vi "test_Read Analog PWM In.vi"(8 "error in (no error)":errorcluster, 11 "TestCase in":refnum<class "FPGA Addon Speciality IO Tests.lvclass">=refnum) -> (0 "error out":errorcluster, 3 "TestCase out":refnum<class "FPGA Addon Speciality IO Tests.lvclass">)   [LabVIEW 2026, in "FPGA Addon Speciality IO Tests.lvclass"]
uses:
  FPGA Addon Speciality IO Tests.lvclass
  FPGA Addon Test Class/FPGA Addon Test Class.lvclass
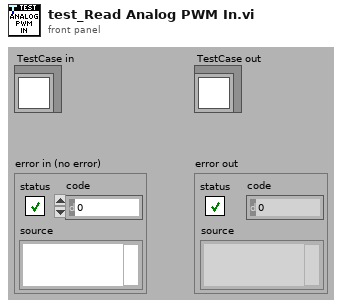
[diagram p1: front panel]
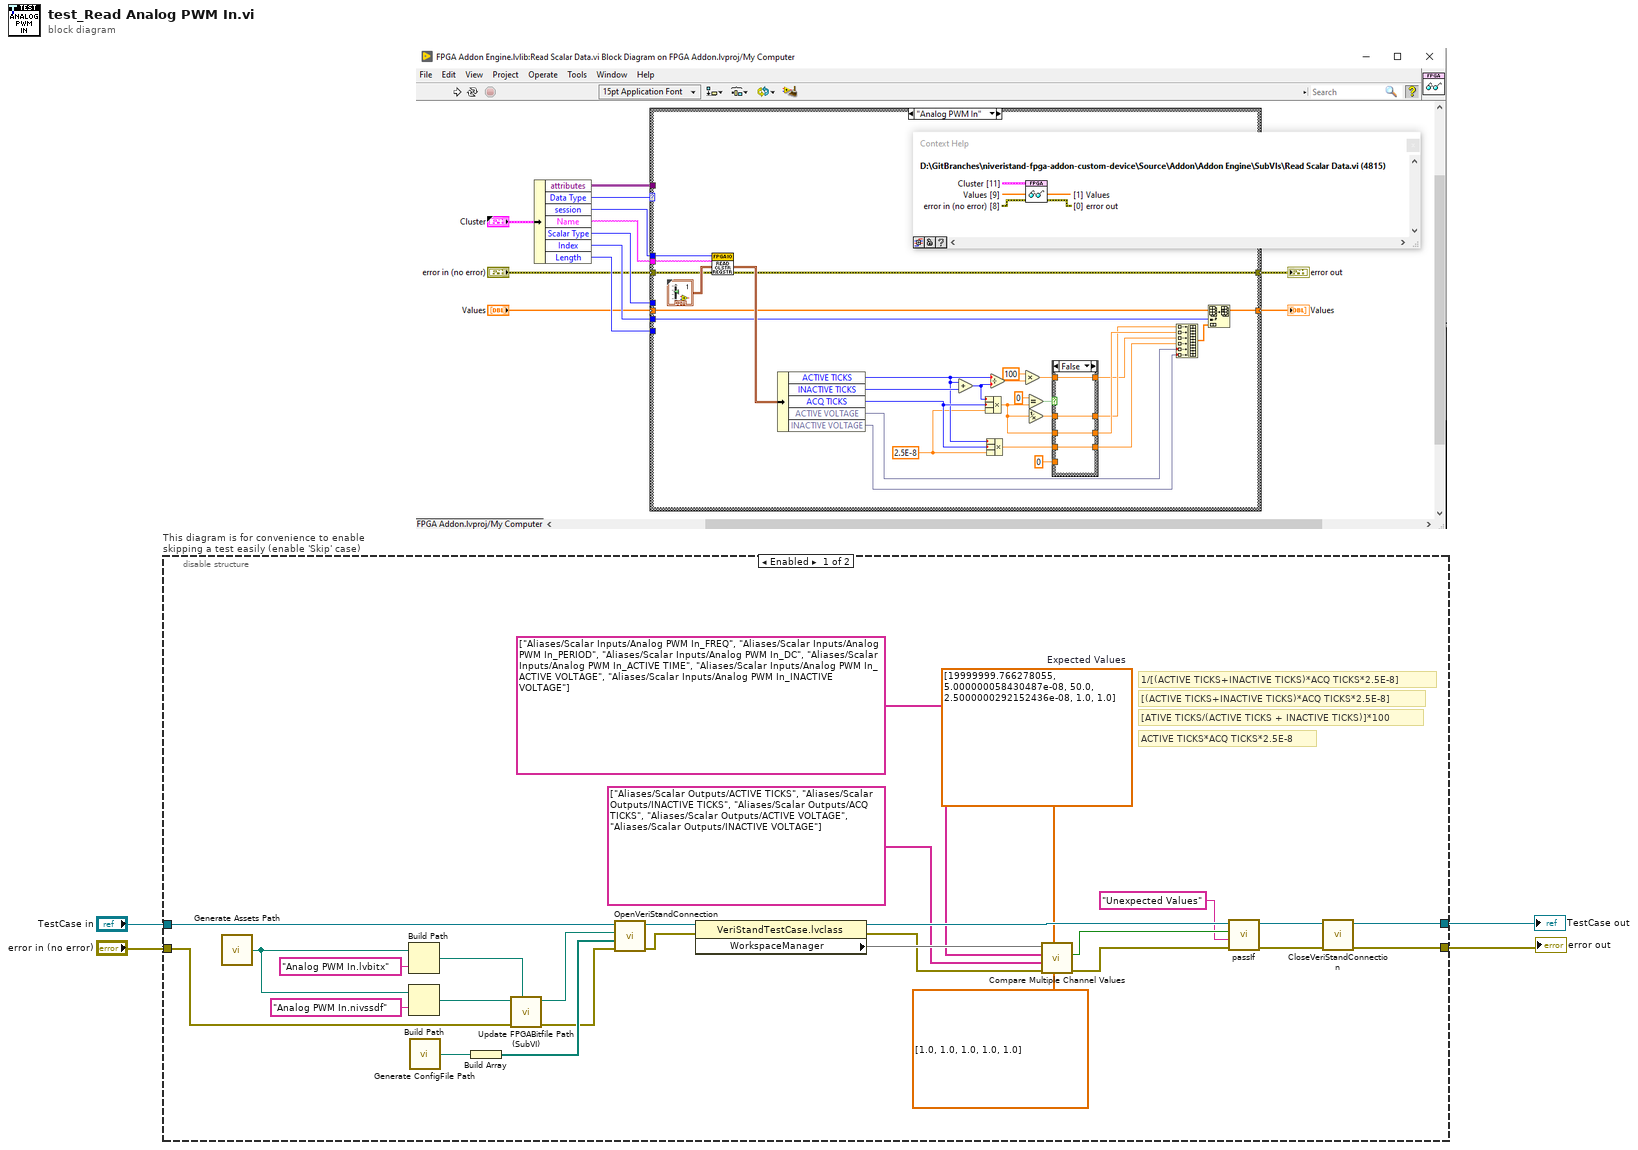
[diagram p0: block diagram]
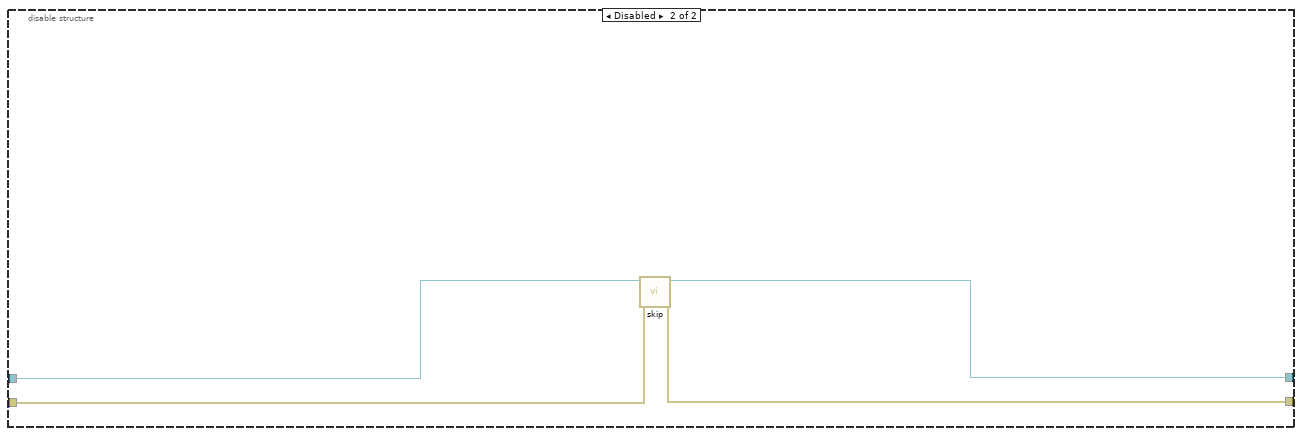
[diagram p2: hidden frame]
diagram:
  n1 = disable-structure "This diagram is for convenience to enable skipping a test easily (enable 'Skip' case)" shown="Enabled" {
    disable-tunnel: "TestCase in" -> [w29 w35]
    disable-tunnel: [w26 w33] -> w1
    disable-tunnel: [w27 w34] -> w3
    disable-tunnel: "error in (no error)" -> [w7 w32]
    frame Enabled {
      w16 = dbl[] [19999999.766278055, 5.000000058430487e-08, 50.0, 2.5000000292152436e-08, 1.0, 1.0]  # Expected Values
      # "ACTIVE TICKS*ACQ TICKS*2.5E-8"
      # "[ATIVE TICKS/(ACTIVE TICKS + INACTIVE TICKS)]*100"
      # "[(ACTIVE TICKS+INACTIVE TICKS)*ACQ TICKS*2.5E-8]"
      # "1/[(ACTIVE TICKS+INACTIVE TICKS)*ACQ TICKS*2.5E-8]"
      n2 = call "Generate Assets Path.vi"() -> ("Assets path"=w12:path)
      n3 = Build Path(base path=w12, name or relative path="Analog PWM In.lvbitx") -> (appended path=w9:path)
      n4 = Build Path(base path=w12, name or relative path="Analog PWM In.nivssdf") -> (appended path=w8:path)
      n5 = call "Generate ConfigFile Path.vi"() -> ("ConfigFile path"=w25:path)
      n6 = Build Array(w25) -> (w28:path[])
      n7 = call "Update FPGABitfile Path (SubVI).vi"("Bitfile Path"=w9, "error in (no error)"=w7, "System Definition path in"=w8) -> ("error out"=w6:errorcluster, "System Definition path out"=w5:path)  [unwired: 7 in]
      n8 = call-dynamic "OpenVeriStandConnection.vi"("error in (no error)"=w6, "overrides files"=w28, "System Definition File"=w5, "VeriStand Test Case in"=w29) -> ("error out"=w31:errorcluster, "VeriStand Test Case out"=w30:refnum<class "VeriStandTestCase.lvclass">)  [unwired: 5 in, 1 out]
      n9 = property class="VeriStandTestCase.lvclass"(reference=w30, error in=w31) -> (reference out=w24:refnum<class "VeriStandTestCase.lvclass">, error out=w20:errorcluster, "WorkspaceManager"=w21)
      n10 = call "Compare Multiple Channel Values.vi"("Values"=dbl[] [1.0, 1.0, 1.0, 1.0, 1.0], "Expected Values"=w16, "error in (no error)"=w20, "Scalar Outputs"=string[] ["Aliases/Scalar Outputs/ACTIVE TICKS", "Aliases/Scalar Outputs/INACTIVE TICKS", "Aliases/Scalar Outputs/ACQ TICKS", "Aliases/Scalar Outputs/ACTIVE VOLTAGE", "Aliases/Scalar Outputs/INACTIVE VOLTAGE"] ("Channels"), "Scalar Inputs"=string[] ["Aliases/Scalar Inputs/Analog PWM In_FREQ", "Aliases/Scalar Inputs/Analog PWM In_PERIOD", "Aliases/Scalar Inputs/Analog PWM In_DC", "Aliases/Scalar Inputs/Analog PWM In_ACTIVE TIME", "Aliases/Scalar Inputs/Analog PWM In_ACTIVE VOLTAGE", "Aliases/Scalar Inputs/Analog PWM In_INACTIVE VOLTAGE"] ("Channels"), ".NET Refnum in"=w21) -> ("error out"=w15:errorcluster, "Equals?"=w14:bool)  [unwired: 4 in]
      n11 = call-dynamic "passIf.vi"("error in (no error)"=w15, "message (\"\")"="Unexpected Values" ("message (\"\")"), "pass"=w14, "TestCase in"=w24) -> ("error out"=w22:errorcluster, "TestCase out"=w23:refnum<class "FPGA Addon Speciality IO Tests.lvclass">)  [unwired: 6 in]
      n12 = call-dynamic "CloseVeriStandConnection.vi"("error in (no error)"=w22, "VeriStand Test Case in"=w23) -> ("error out"=w27:errorcluster, "VeriStand Test Case out"=w26:refnum<class "VeriStandTestCase.lvclass">)  [unwired: 8 in]
    }
    frame Disabled {
      # "skip test result while test is under development"
      n13 = call <vilib>:"skip.vi"("error in (no error)"=w32, "TestCase in"=w35) -> ("error out"=w34:errorcluster, "TestCase out"=w33:refnum<class "FPGA Addon Speciality IO Tests.lvclass">)  [unwired: 8 in]
    }
  }
  "error out" <- w3
  "TestCase out" <- w1
